vi "RelU Vector Elements.vi"(2 "X":T1) -> (16 "RelU(X)":T1)   [LabVIEW 2014]
uses:
  <vilib>/Analysis/Matrix/Datatypes/RealMatrix.ctl
  <vilib>/Analysis/Matrix/NI_Matrix.lvlib
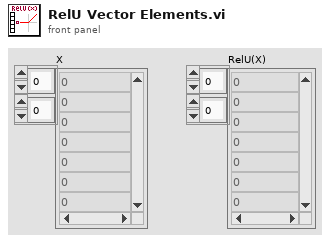
[diagram p1: front panel]
types:
  T1 = typedef "NI_Matrix.lvlib/RealMatrix.ctl" = dbl[][]
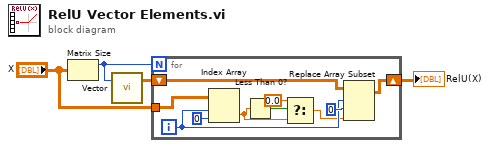
[diagram p0: block diagram]
diagram:
  n1 = Matrix Size(0:"X") -> (1:w3:i32)  [unwired: 1 out]
  n2 = call "Vector.vi"("length"=w3) -> ("Real Matrix (Column Vector)"=w2:T1)  [unwired: 18 in]
  n3 = for {
    N: w3 -> [_]
    tunnel: "X" -> [w11]
    shift-right: [w13] -> w1
    shift-left: w2 -> [w14]
    i -> [w10]
    n4 = Index Array(array=w11, index (row)=w10, index (col)=0) -> (element=w6:dbl)
    n5 = Less Than 0?(x=w6) -> (x < 0?=w7:bool)
    n6 = Select(t=0.0, s=w7, f=w6) -> (s? t:f=w5:dbl)
    n7 = Replace Array Subset(array=w14, new element=w5, index (row)=w10, index (col)=0 ("disabled index (col)")) -> (w13:T1)
  }
  "RelU(X)" <- w1
